vi "Unregister API.vi"(8 "error in (no error)":errorcluster, 10 "API":refnum<class "API.lvclass">, 11 "VolatusCore in":refnum<class "VolatusCore.lvclass">) -> (0 "error out":errorcluster, 3 "VolatusCore out":refnum<class "VolatusCore.lvclass">)   [LabVIEW 2020, in "Volatus.lvlib" / "VolatusCore.lvclass"]
uses:
  VolatusCore.lvclass
  VolatusCore.lvclass/VolatusCore.ctl
  Identity/Identity.lvclass
  API/API.lvclass
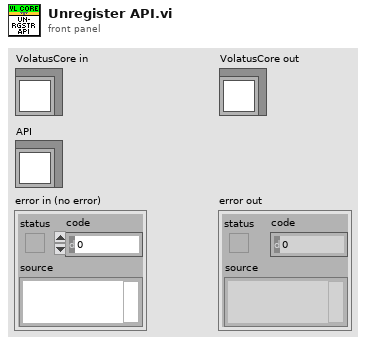
[diagram p1: front panel]
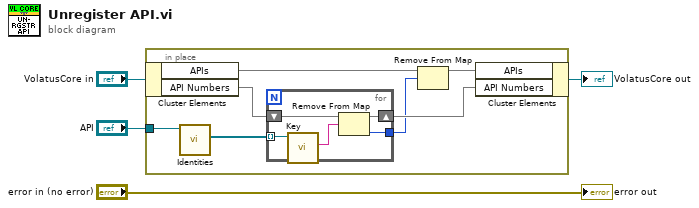
[diagram p0: block diagram]
diagram:
  n1 = in-place {
    in-place-border: "API" -> [w11]
    n2 = in-place-cluster #1("VolatusCore in") -> ("APIs"=w7:map{u32, refnum<class "API.lvclass">}, "API Numbers"=w9:map{string, u32})
    n3 = call-dynamic "Identities.vi"("API in"=w11) -> ("Identities"=w10:refnum<class "Identity.lvclass">[])  [unwired: 8 in, 2 out]
    n4 = for {
      tunnel: w10 -> [w16] mode=indexing
      shift-right: [w13] -> w8
      shift-left: w9 -> [w15]
      tunnel: [w12] -> w5
      n5 = call "Key.vi"("Identity in"=w16) -> ("Key"=w14:string)  [unwired: 10 in]
      n6 = Remove From Map(10:w14, 11:w15) -> (1:w12:u32, 3:w13:map{string, u32})  [unwired: 1 out]
    }
    n7 = Remove From Map(10:w5, 11:w7) -> (3:w6:map{u32, refnum<class "API.lvclass">})  [unwired: 2 out]
    n8 = in-place-cluster #1("APIs"=w6, "API Numbers"=w8) -> (→"VolatusCore out":refnum<class "VolatusCore.lvclass">)
  }
  "error out" <- "error in (no error)"
